vi "tearDown.vi"(8 "error in (no error)":errorcluster, 11 "reference in":refnum<class "Test Numeric Test Object.lvclass">) -> (0 "error out":errorcluster, 3 "reference out":refnum<class "Test Numeric Test Object.lvclass">)   [LabVIEW 2009, in "Test Numeric Test Object.lvclass"]
doc: "tearDown runs after the test method has completed. Use this method to clean up any operations or references that were opened by setUp or the test method. Unit tests should be independent of other unit tests so this VI should ensure that the next test can run in a 'clean' test environment."
uses:
  Test Numeric Test Object.lvclass
  Test Numeric Test Object.lvclass/Test Numeric Test Object.ctl
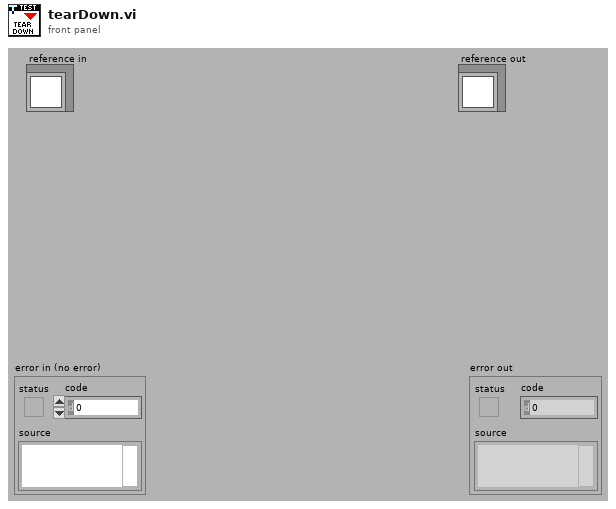
[diagram p1: front panel]
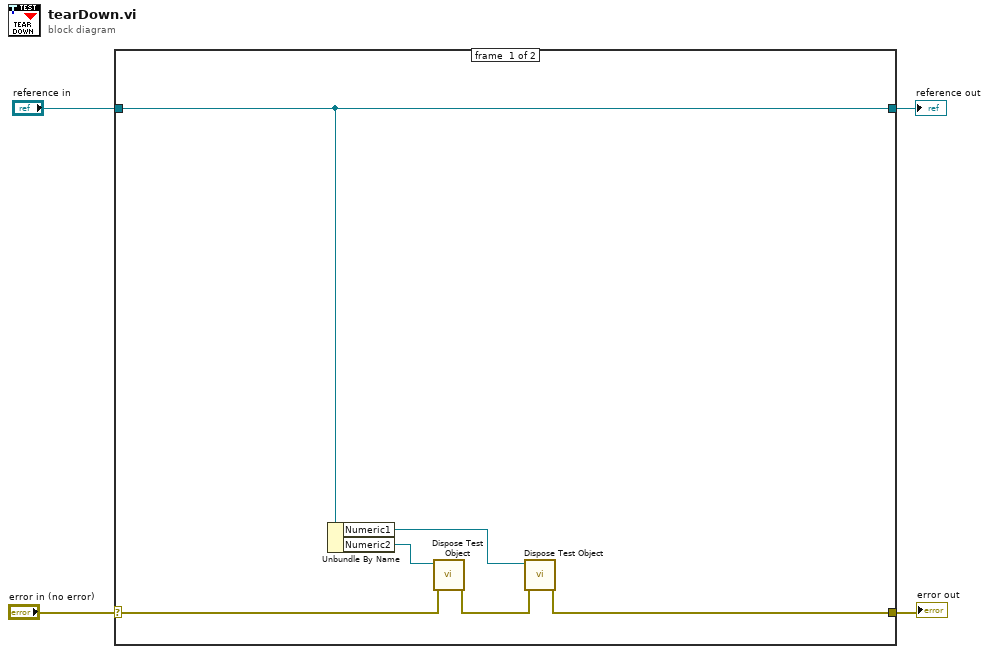
[diagram p0: block diagram]
diagram:
  n1 = case shown="No Error" "error in (no error)" {
    selector: "error in (no error)" -> [w6 w12]
    tunnel: [w8 w12] -> w3
    tunnel: [w10 w11] -> w1
    tunnel: "reference in" -> [w10 w11]
    frame #0 {
      n2 = Unbundle By Name(w10) -> ("Numeric1"=w9:refnum<class "Numeric Test Object.lvclass">, "Numeric2"=w7:refnum<class "Numeric Test Object.lvclass">)
      n3 = call "Dispose Test Object.vi"("error in (no error)"=w6, "Numeric"=w7) -> ("error out"=w5:errorcluster)  [unwired: 9 in]
      n4 = call "Dispose Test Object.vi"("error in (no error)"=w5, "Numeric"=w9) -> ("error out"=w8:errorcluster)  [unwired: 9 in]
    }
    frame #1 {
    }
  }
  "error out" <- w3
  "reference out" <- w1
